vi "NotchFilterExample.vi"() -> ()   [LabVIEW 2011]
uses:
  <vilib>/addons/Digital Filter Design/_Objects.llb/DFD Filter Obj.ctl
  <vilib>/addons/Digital Filter Design/_Objects.llb/DFD Filter Coef.ctl
  <vilib>/addons/Digital Filter Design/_Objects.llb/DFD Filter Structure Type Selector.ctl
  <vilib>/addons/Digital Filter Design/_Objects.llb/dfd_Internal Quantization Settings.ctl
  <vilib>/addons/Digital Filter Design/_Objects.llb/dfd_Internal Quantization Srcs.ctl
  <vilib>/addons/Digital Filter Design/_Objects.llb/DFD Coef Norm Type.ctl
  <vilib>/Platform/TimedLoop/XDataNode/timing_clust.ctl
  <vilib>/Platform/TimedLoop/XDataNode/nitl_modes.ctl
  <vilib>/Platform/TimedLoop/XDataNode/wakeup.ctl
  <vilib>/addons/Digital Filter Design/Process.llb/DFD Filtering (PtByPt).vi
  <vilib>/addons/Digital Filter Design/Design.llb/DFD IIR Notch Peak Design by Q.vi
  <vilib>/measure/maspectr.llb/FFT Spectrum (Mag-Phase) for 1 Chan.vi
  <vilib>/Platform/TimedLoop/XDataNode/XDataNode.xnode
  <vilib>/addons/Digital Filter Design/NI_DigFilterLicensed.lvlib
  <vilib>/Platform/TimedLoop/XDataNode/XDNodeRunTimeDep.lvlib
  <vilib>/measure/NI_MAPro.lvlib
  <vilib>/Analysis/NI_AAL_SigProc.lvlib
panel:
  out "Waveform Graph":cluster{"f0":dbl, "df":dbl, "magnitude":dbl[]}(graph)
  out "Spectrum":T1(graph)={"magnitude"={"f0"=0.0, "df"=0.5, "magnitude"=array[500 elements]}, {"Locations"=[], "Amplitudes"=[]}}
  out "Peaks":cluster{"Locations":dbl[], "Amplitudes":dbl[]}
  out "FFTArray":dbl[](array[numeric])=[-5.97568735222049, -5.621732107397926, -5.038552645886518, -4.450468686097488, -4.0821691176339865, -4.0728882671460385, -4.423228798393417, -4.994943068826768, -5.563756411436293, -5.905055575012764, -5.8797121598680775, -5.4872592999993826, -4.866109771074623, -4.240732057590185, -3.8359611486272436, -3.791174228170831, -4.107113012463757, -4.6456645588715375, -5.182684017201283, -5.4936825586907805, -5.439650321745023, -5.020232627328567, -4.373947645235918, -3.7253620463457016, -3.2994014118795763, -3.2355255672229566, -3.53455059410871, -4.058429346991616, -4.583073945645599, -4.884043480291713, -4.822366769137059, -4.397718422044574, -3.7486363921120525, -3.0996975507319715, -2.67582805745418, -2.616478692364337, -2.9224469047901422, -3.455657403996944, -3.991984763648453, -4.3069412758428225, -4.2614998940832125, -3.855270518111671, -3.2267178015449245, -2.600337016849979, -2.2009647478759327, -2.167954576318933, -2.501999514596405, -3.0649130092321335, -3.632451984924015, -3.9800051633614593, -3.9684164942971876, -3.5971619499191885, -3.0045678614038747, -2.414987330139949, -2.053111481635458, -2.058145726336352, -2.430632777490008, -3.032234247915363, -3.63855429344588, -4.024828534809719, -4.051748093021613, -3.7186369869648788, -3.1636710696775863, -2.6110550334332903, -2.285334249334319, -2.3255716032657636, -2.732171076147873, -3.366659888069586, -4.004512671954646, -4.420840906380969, -4.476217440679121, -4.169854358986797, -3.639822357984511, -3.1102281666274734, -2.8055267719761563, -2.8646986114404758, -3.288073477970472, -3.93711295649828, -4.587234856114255, -5.013502866617332, -5.076451271616947, -4.775262964201894, -4.247988939226518, -3.7187257901481385, -3.411927974143003, -3.4665850057353715, -3.8830453254033332, -4.5227986616527796, -5.1613003513183635, -5.573660847179018, -5.6204702456554125, -5.30097608132646, -4.753302563210926, -4.2016277817257155, -3.8704956512435382, -3.898992749691152, -4.287571803114556, -4.897833635176491, -5.505351048003509, -5.8853578651631215, -5.8985729714374155, -5.544377597989529, -4.961034029931568, -4.372862267260028, -4.004551406249719, -3.9953359049822654, -4.3458184831566875, -4.917751478503985, -5.4868601285243965, -5.828531010742922, -5.8036354784589035, -5.411706343049822, -4.7911559821472816, -4.166452407081848, -3.7624300589685347, -3.7184654994695663, -4.035299748633417, -4.574819094338727, -5.112877844252291, -5.424986255538461, -5.372133481384279, -4.953963787254436, -4.308994218095225, -3.6617902515812126, -3.237276208462303, -3.1749105875042387, -3.475508078894869, -4.001020081877478, -4.527357198700525, -4.830076941127196, -4.770206489455651, -4.347418757702761, -3.700249946768749, -3.0532751211403877, -2.6314185804511787, -2.574129193616205, -2.8822024493396947, -3.4175610486766876, -3.9560775113904016, -4.273262031963773, -4.230085424554836, -3.8261554098870962, -3.1999344249714836, -2.575915490221136, -2.178932904134167, -2.1483379319809455, -2.4848212409065553, -3.050193905593625, -3.6202104546267977, -3.9702571916339395, -3.9611756287252606, -3.592439283228705, -3.0023720166497556, -2.4153244482992204, -2.0559852116514357, -2.0635572175870505, -2.438580674730889, -3.0427146886731977, -3.651560907900572, -4.040352448138856, -4.069777930226654, -3.739158880178784, -3.1866686679385774, -2.6365095149383793, -2.313224336133132, -2.355873578424281, -2.764858803333255, -3.401704833564521, -4.041883929062132, -4.460505222229892, -4.518139245370435, -4.213995797085913, -3.6861433223131272, -3.158686334338146, -2.856077642869327, -2.9172955484921985, -3.3426677500351385, -3.993653783142716, -4.645669454557922, -5.073776500704439, -5.138507302816345, -4.839042904548417, -4.3134325061869365, -3.785770963328159, -3.4805110538215676, -3.5366406731292472, -3.9545067046380984, -4.595597383365241, -5.235366617833823, -5.64892349920171, -5.696856830407549, -5.378412922075821, -4.831714830110095, -4.280939563913337, -3.9506300301078467, -3.979871873262168, -4.3691169614859104, -4.979965336896743, -5.5879890973503015, -5.9684214402525715, -5.98198070305598, -5.628047649102335, -5.044884175770395, -4.456809975924332, -4.08851391974228, -4.079230320581869, -4.429561835075211, -5.001260819724555, -5.570052612762078, -5.91132397441526, -5.885946522626465, -5.493453415206553, -4.872257457812066, -4.246827171079447, -3.8419975863494646, -3.7971459359695063, -4.11301399059333, -4.651488868014997, -5.188425784421577, -5.499335983347278, -5.445209681325951, -5.025692283231612, -4.379302048467413, -3.7306057431427964, -3.3045290492455734, -3.240531898371193, -3.539430483814445, -4.063177776836101, -4.587686019162704, -4.888514427985717, -4.826691953399974, -4.40189334194204, -3.752656688045358, -3.1035590089586815, -2.679526614489999, -2.620010439224742, -2.9258080910978457, -3.4588444419327233, -3.9949942317513787, -4.309769922651276, -4.264144641613878, -3.857728465171484, -3.2289862268718275, -2.602413382091327, -2.202846700372251, -2.169639951728965, -2.5034863393238003, -3.066199502682131, -3.6335365615561814, -3.980886434568021, -3.969093270084828, -3.5976332403932267, -3.00483287806273, -2.415045486969899, -2.0529623960081724, -2.057789219704304, -2.4300688758869358, -3.0314631822482, -3.637576499596384, -4.02364465351577, -4.050358969573484, -3.7170436706902104, -3.161874813225746, -2.60905729185776, -2.2831366789737193, -2.32317606042377, -2.7295796155764096, -3.363874761248236, -4.001536325176325, -4.417675978648588, -4.472866761392593, -4.166320945455444, -3.63610941273502, -3.106339074542322, -2.8014650972255586, -2.8604680942534175, -3.2836780312128524, -3.932556662080569, -4.582521961225087, -5.008637779789445, -5.071438558628105, -4.770107343809544, -4.242695278751824, -3.713299100894393, -3.4063734066835916, -3.460907845037558, -3.8772509858228417, -4.51689268178706, -5.155288388739395, -5.567548673021065, -5.614263739102609, -5.294681223971307, -4.746925433311064, -4.195174548350359, -3.8639725683239186, -3.8924061499761455, -4.280928092041427, -4.891139284660897, -5.498612590144155, -5.878581885895967, -5.891766104105767, -5.537546516874269, -4.9541854437162955, -4.366002912468052, -3.9976880406290696, -3.9884753008638563, -4.338967420792041, -4.9109167393786475, -5.4800484886628205, -5.821749234007299, -5.796890309851494, -5.405004502018551, -4.784504155913032, -4.159857243975239, -3.7558981618133718, -3.7120034189824933, -4.028913976874615, -4.568516058206815, -5.106663899035053, -5.418867678523341, -5.366116465536588, -4.948054434966055, -4.303198535018516, -3.656114140544593, -3.2317254634732495, -3.1694908878642893, -3.4702249834036305, -3.995879023159046, -4.522363477630227, -4.82523572140044, -4.765522792262976, -4.342897456551172, -3.6958957624356126, -3.049092616770561, -2.627412156802884, -2.5703030844570156, -2.87856071700568, -3.4141075797874505, -3.9528160127409544, -4.270196026570565, -4.2272182478951335, -3.823490206307066, -3.1974741442826664, -2.57366288447373, -2.1768905245989174, -2.1465081263058363, -2.483206150482008, -3.0487954631102827, -3.6190303818404144, -3.9692969973331236, -3.9604366069070593, -3.591922511482165, -3.002078354748901, -2.4152545370194805, -2.0561394717812216, -2.063935849176584, -2.439183656540288, -3.0435417778527367, -3.652611639873718, -4.041626136717718, -4.071273667942322, -3.740875538825938, -3.188604899345653, -2.6386637519522402, -2.3155947938232346, -2.358458255500911, -2.767655483787516, -3.4047110885148753, -4.0450971188268685, -4.463922498592392, -4.521757554071387, -4.217811880513517, -3.690153722402035, -3.162887395668834, -2.8604655159682792, -2.92186619332818, -3.34741693971202, -3.998577107777304, -4.650762325347665, -5.079034154185074, -5.143924805282298, -4.844615156665586, -4.319154247761323, -3.791636778258488, -3.486515375191596, -3.5427777884791163, -3.960770761371564, -4.601982394311398, -5.241866466948132, -5.655531947404552, -5.703567521554442, -5.385219389047899, -4.838610501030982, -4.287917768467314, -3.9576840059840306, -3.9869947726809474, -4.376301857830287, -4.987205231427335, -5.5952769260115325, -5.975750080536178, -5.989342980951666, -5.635436346098064, -5.052292035915185, -4.464229712933551, -4.095938224146738, -4.086651866909996, -4.436973289063696, -5.008654845550782, -5.577421880278855, -5.9186611664110185, -5.8932443420617195, -5.5007045924602895, -4.879454757897257, -4.253963400851944, -3.8490656016727236, -3.8041386488467386, -4.119924376259602, -4.658309971972454, -5.195150729418968, -5.505957976294024, -5.451722020134827, -5.032088363578573, -4.385575370471935, -3.7367499179437997, -3.310537805496792, -3.246399088612273, -3.545150090739972, -4.068743919441895, -4.593092958769223, -4.893756574130159, -4.831763869590888, -4.406789751268074, -3.757372478641705, -3.1080892393151047, -2.683866518592444, -2.6241554315480444, -2.929753771410782, -3.4625865999425915, -3.9985288515506543, -4.313093187001207, -4.267252936017326, -3.86061838176643, -3.2316545681211744, -2.6048571642713734, -2.2050631568561982, -2.171626536058367, -2.505240728073047, -3.067719598099761, -3.634820493999401, -3.981932564696965, -3.9699001908512184, -3.5981997787931608, -3.0051580966650997, -2.4151286852051976, -2.05280311124362, -2.057387228066914, -2.429424192864066, -3.0305760630449603, -3.636447439263071, -4.02227438683535, -4.048748470713145, -3.7151941526149286, -3.159787726873427, -2.6067343250881154, -2.2805797552619365, -2.3203873373422974, -2.7265614830242386, -3.360629839462558, -3.998067462499014, -4.4139862490763075, -4.468959461896693, -4.162199593072044, -3.6317777414407986, -3.1018010319062332, -2.7967248408464696, -2.855529987981699, -3.2785466411679898, -3.9272367524553355, -4.577018489899442, -5.002955893727491, -5.065583589099471, -4.764084801410969, -4.236510848247818, -3.7069586358754965, -3.399882924050603, -3.4542735193150205, -3.8704791433107615, -4.509989794548131, -5.148261068436077, -5.560403664611494, -5.607007914379096, -5.287321574979713, -4.7394690656276595, -4.187628674252066, -3.856344499821118, -3.884703291757965, -4.2731579343022466, -4.883309395838602, -5.4907306095679065, -5.870655516352556, -5.883803104333697, -5.5295546939854905, -4.94617264556551, -4.357977019957975, -3.98965695998956, -3.9804469558757862, -4.33094974499072, -4.902917668231767, -5.472075951743317, -5.813811147141563, -5.788994567287549, -5.397158968591169, -4.7767166592335935, -4.152135566639196, -3.7482500336439486, -3.7044365093125826, -4.021435886877789, -4.5611343132853746, -5.099385941260222, -5.411700859166119, -5.359068037653094, -4.941131546087548, -4.296408219919485, -3.6494633141250787, -3.22522091373631, -3.1631392690112645, -3.4640328090551007, -3.9898526596983963, -4.516509137684786, -4.819559457464254, -4.760030490468245, -4.337594830590808, -3.6907883476526084, -3.044185764403578, -2.6227110284212056, -2.565812646558062, -2.8742857358047464, -3.410052616195501, -3.9489854175373282, -4.266593935775643, -4.223848578348389, -3.8203566514517924, -3.194580170170159, -2.5710117259822614, -2.174485181869182, -2.1443513614181446, -2.481300484346546, -3.047143172605582, -3.6176334971707047, -3.96815729964722, -3.959555626137596, -3.5913015244452877, -3.0017183834839827, -2.4151563473790807, -2.0563035722724505, -2.064362490052009, -2.4398728291481406, -3.0444932142344032, -3.6538248126286494, -4.043100259105718, -4.0730076942598314, -3.742868165030517, -3.1908545639392134, -2.6411686371114507, -2.318352826802215, -2.361467110270621, -2.7709125829383634, -3.4082136054039247, -4.048841979980092, -4.467906386351882, -4.525976909488011, -4.222262906483061, -3.694832387037704, -3.1677894359227032, -2.865586441466155, -2.9272012904587474, -3.352961275923062, -4.004325536110784, -4.6567094891773175, -5.085174492182694, -5.150252556589672, -4.851124366266319, -4.325838772060686, -3.7984902908534193, -3.4935313728314927, -3.5499495972097552, -3.9680915428608214, -4.609445152340919, -5.249464054082875, -5.663257071803423, -5.7114127539526, -5.393177169875848, -4.8466731476768885, -4.296077482670671, -3.9659328813559305, -3.995324802342266, -4.384704942163973, -4.995673185928899, -5.603801489239893, -5.984322922157577, -5.997955709850103, -5.644080518574551, -5.060959163937324, -4.472911272459232, -4.104625663474488, -4.095336615091996, -4.445646764334581, -5.017308463788067, -5.586047063477411, -5.927249351164297, -5.901786988044713, -5.509193190897225, -4.8878808400194655, -4.262318546316348, -3.8573414469655356, -3.812326895626229, -4.128016799655316, -4.666298428822866, -5.203027166449752, -5.513714438202357, -5.459350657608405, -5.039581441210377, -4.392925274583408, -3.7439491642923217, -3.3175790468723445, -3.253275122308536, -3.551853865896033, -4.07526854424731, -4.599431707512776, -4.899902894114951, -4.8377113878678655, -4.412532281220043, -3.7629040263799887, -3.1134040099098668, -2.688958922104338, -2.6290200888701403, -2.9343855199168543, -3.4669804989229025, -4.002680187441947, -4.316997478398468, -4.270905938467135, -3.8640160923280105, -3.234793229704079, -2.607733269724446, -2.207673452834965, -2.1739680266301677, -2.507310678082698, -3.0695155362803326, -3.6363402158282607, -3.9831741349923915, -3.9708619461077195, -3.5988803292493037, -3.0055563281097992, -2.4152437605105157, -2.052634471621743, -2.05693459406838, -2.4286875650855086, -3.0295557225761476, -3.6351439478399756, -4.020688586738384, -4.046881484366051, -3.713047381922518, -3.1573628522749733, -2.6040333043349344, -2.277604821921041, -2.317140999021156, -2.7230465193284084, -3.356849299673936, -3.994024662996037, -4.409684770467747, -4.464403145907171, -4.157392539157608, -3.6267243031464567, -3.0965058129578074, -2.7911926910082596, -2.8497659986459287, -3.2725561407097237, -3.921025301338388, -4.570591875553075, -4.996320125185829, -5.05874489141586, -4.757049609847138, -4.229285802251864, -3.699550572844767, -3.3922988728836456, -3.446520693780551, -3.862564935205337, -4.50192176668307, -5.140046947428074, -5.552051333514287, -5.598525405144494, -5.278717060755513, -4.730750852909591, -4.178805194888971, -3.8474243028842556, -3.8756950352801813, -4.264070376900983, -4.874151388219596, -5.481511085936418, -5.8613834857098635, -5.874487641704263, -5.5202049315558455, -4.936797763754813, -4.348586238426562, -3.9802595285947824, -3.97105214558322, -4.321566838752948, -4.893555951835543, -5.462744704643959, -5.80451963329307, -5.779752025960149, -5.387974605214614, -4.767599636244794, -4.143094994375555, -3.739294961251586, -3.695575915723579, -4.012678671824875, -4.552489288389496, -5.090861821189817, -5.403306252876029, -5.350811439718738, -4.933021328131873, -4.288452622155449, -3.64167043700269, -3.2175987097330863, -3.155695534538873, -3.4567751765143084, -3.982788589682157, -4.509645911346777, -4.8129041690346686, -4.753590039961196, -4.331375916679908, -3.684797460742717, -3.0384291798894814, -2.6171948001528618, -2.560542600512994, -2.869267463977555, -3.4052914707033497, -3.944486504958051, -4.262362111724113, -4.219888442276495, -3.8166725417110077, -3.191176159309315, -2.5678916163153285, -2.171652501290262, -2.141809359484656, -2.47905212863597, -3.0451911453384284, -3.6159801921137626, -3.966804819295521, -3.9585057791819533, -3.590555823520937, -3.001278043215203, -2.4150222827031866, -2.056476397075878, -2.064842516083454, -2.4406600652373176, -3.0455873658074033, -3.6552252815218034, -4.044806143679235, -4.075017789811855, -3.7451809645083003, -3.1934682589557517, -2.644081119256466, -2.3215616892483006, -2.364969649689641, -2.7747058016973885, -3.4122942140715806, -4.053206400105752, -4.472550753557612, -4.530897076825501, -4.227454448091083, -3.7002906020735984, -3.1735093527719878, -2.8715628222288925, -2.933428635701005, -3.3594338297011093, -4.011037291249605, -4.663654192810659, -5.0923456515418986, -5.157643445038536, -4.858728029578418, -4.333648034930868, -3.806497763629879, -3.501729458488085, -3.55833049851534, -3.976647269769748, -4.618167529577204, -5.258344728926826, -5.672287522061034, -5.72058429610693, -5.402480967407508, -4.8561002195543015, -4.305618711992345, -3.975579024135332, -4.005066496447421, -4.394532716370502, -5.005577469109998, -5.613772619653975, -5.994351156853354, -6.008031234162517, -5.654193455702178, -5.071099584601804, -4.483069204628833, -4.114791102146382, -4.105499532119519, -4.455797118298613, -5.02743620988949, -5.596142163460768, -5.937301783231151, -5.911786756785091, -5.519130337201699, -4.897745450971697, -4.272100765056629, -3.8670314825139074, -3.821915032655541, -4.1374934082077734, -4.6756539739517695, -5.2122522177876665, -5.5227996794437555, -5.468286895882232, -5.048359616360676, -4.401536468318877, -3.752384609227775, -3.3258301354130193, -3.261333415413767, -3.559711101671834, -4.082916646386913, -4.606862793565731, -4.907109283575152, -4.844685610079926, -4.4192670830840335, -3.7693923798592297, -3.1196391193253943, -2.6949342312116835, -2.6347292877118065, -2.939822551440289, -3.4721395653593774, -4.007555756447308, -4.321584288924292, -4.275199006390161, -3.868010715804723, -3.238484994261437, -2.611118053069307, -2.210747429385189, -2.1767276717592328, -2.509752772075492, -3.0716371679895413, -3.6381387860353214, -3.9846473594706087, -3.972007858364352, -3.59969728297488, -3.0060429993000004, -2.4153991492892866, -2.052457903732966, -2.056425722052905, -2.4278463691412373, -3.0283825110907063, -3.6336393576025925, -4.018853582826432, -4.044717359710772, -3.710555756543763, -3.154545672199507, -2.6008928401790263, -2.2741436671689947, -2.3133620679642286, -2.718953044691952, -3.352444829926184, -3.9893130593393855, -4.404670203516313, -4.459090092055842, -4.151785776638609, -3.6208289077881464, -3.0903271536385093, -2.7847364248089512, -2.8430380657250605, -3.2655627588731146, -3.9137729603433873, -4.563087331115283, -4.988570392737175, -5.050757239572912, -4.74883155363896, -4.220845096076847, -3.690895203197259, -3.383437050825514, -3.4374608471836794, -3.8533157007721766, -4.492491981741846, -5.130445641521714, -5.542287719783991, -5.588608871518526, -5.268657160952961, -4.720557297266353, -4.168487841006326, -3.836993146135313, -3.865160199146582, -4.253442103179915, -4.863440027090745, -5.470727085912743, -5.850537383471874, -5.863590051832546, -5.5092665361680115, -4.925829302064603, -4.337598496226178, -3.969263327670066, -3.960058333090827, -4.310586276539543, -4.882599505740745, -5.451823233765801, -5.793643979257983, -5.768933002188373, -5.377222986193022, -4.7569261468257755, -4.132510299106359, -3.728809653747007, -3.6852005080893075, -4.002423584150208, -4.542364838307881, -5.080878213534376, -5.3934735694132305, -5.341139629004578, -4.923520195475749, -4.279131819709457, -3.632539453988619, -3.208666862813941, -3.1469719583453366, -3.4482688143389457, -3.974508184342159, -4.501599996237134, -4.805101059369049, -4.746037824217132, -4.324082448255902, -3.6777703498249843, -3.0316757855645227, -2.6107222227324143, -2.5543576741248213, -2.8633767493898525, -3.399701248422441, -3.9392027685767923, -4.257390561555547, -4.2152344792644305, -3.812341261621601, -3.1871723472206854, -2.564219741402525, -2.16831671191447, -2.138813478592101, -2.4763996494699243, -3.042885227469357, -3.614023657801723, -3.9652001501612086, -3.9572551132284013, -3.589660952477597, -3.0007404102273916, -2.4148429803563762, -2.0566561657660607, -2.0653817427316, -2.441558782353785, -3.046845250899329, -3.656841656854458, -4.046779976392003, -4.077347692371797, -3.7478651955301725, -3.196504724357843, -2.6474673737838823, -2.3252949383300954, -2.3690467516490394, -2.7791232703123723, -3.417048221474208, -4.0582927800265045, -4.47796500490699, -4.536634367616659, -4.233509619687866, -3.706658173776228, -3.180183526715912, -2.8785374886233335, -2.9406973783658517, -3.366989931923136, -4.018873741943371, -4.671763692986944, -5.100720621052456, -5.1662760296299375, -4.867610108213487, -4.342771227393865, -3.815853438392654, -3.5113087408417716, -3.5681242789522942, -3.9866462126102125, -4.6283620818400975, -5.268725129412937, -5.6828438106784125, -5.731306323384437, -5.413358404229662, -4.867122567072562, -4.316775311735933, -3.9868590682825973, -4.016459038264088, -4.406026680806378, -5.017161663533356, -5.625435744721792, -6.006081817503519]
  in  "ChartLength":dbl=2000.0
  out "Notch":T2={"mSRate_Fs"=1000.0, "mSRate_Version"="2.0", "mSRate_Comments"="", "mSRate_OrgCoef"={"type"=enum."IIR Direct Form II", "gain"=1.0, "coef a (k)"=[1.0, -1.9974443312996026, 0.9984304360830942], "coef b (v)"=[0.9992152180415471, -1.9974443312996026, 0.9992152180415471]}, "mSRate_CurCoef"={"type"=enum."IIR Direct Form II", "gain"=1.0, "coef a (k)"=[1.0, -1.9974443312996026, 0.9984304360830942], "coef b (v)"=[0.9992152180415471, -1.9974443312996026, 0.9992152180415471]}, "mSRate_Quantized?"=FALSE, "mSRate_QCoef"={"type"=enum."Undefined", "gain"=1.0, "coef a (k)"=[], "coef b (v)"=[]}, "mSRate_QSettings"=[], "mSRate_Order"=2, "mSRate_Scaling"={"mSRate_ScaleByPowerOf2?"=FALSE, "mSRate_ScaleType"=enum."No Norm"}} {"mSRate_QSettings"."source" items=["Coef a/k"=0, "Coef b/v"=7, "Input"=1, "Output"=2, "Multiplicand"=3, "Product"=4, "Sum"=5, "Delay"=6, "Gain"=8]}
  in  "Q":dbl=20.0 format="%.2f"
  in  "SigFreq(Hz)":dbl=10.0
  out "Finished Late? [i-1]":bool
  out "Waveform Chart":cluster{dbl, "signal out":dbl}(graph)={-1.943171217609549, "signal out"=-5.97568735222049}
  in  "stop":bool
  in  "NotchFreq(Hz)":dbl=5.0 format="%.2f"
  in  "LoopFreq(Hz)":dbl=1000.0 caption="Set Loop Period (us)"
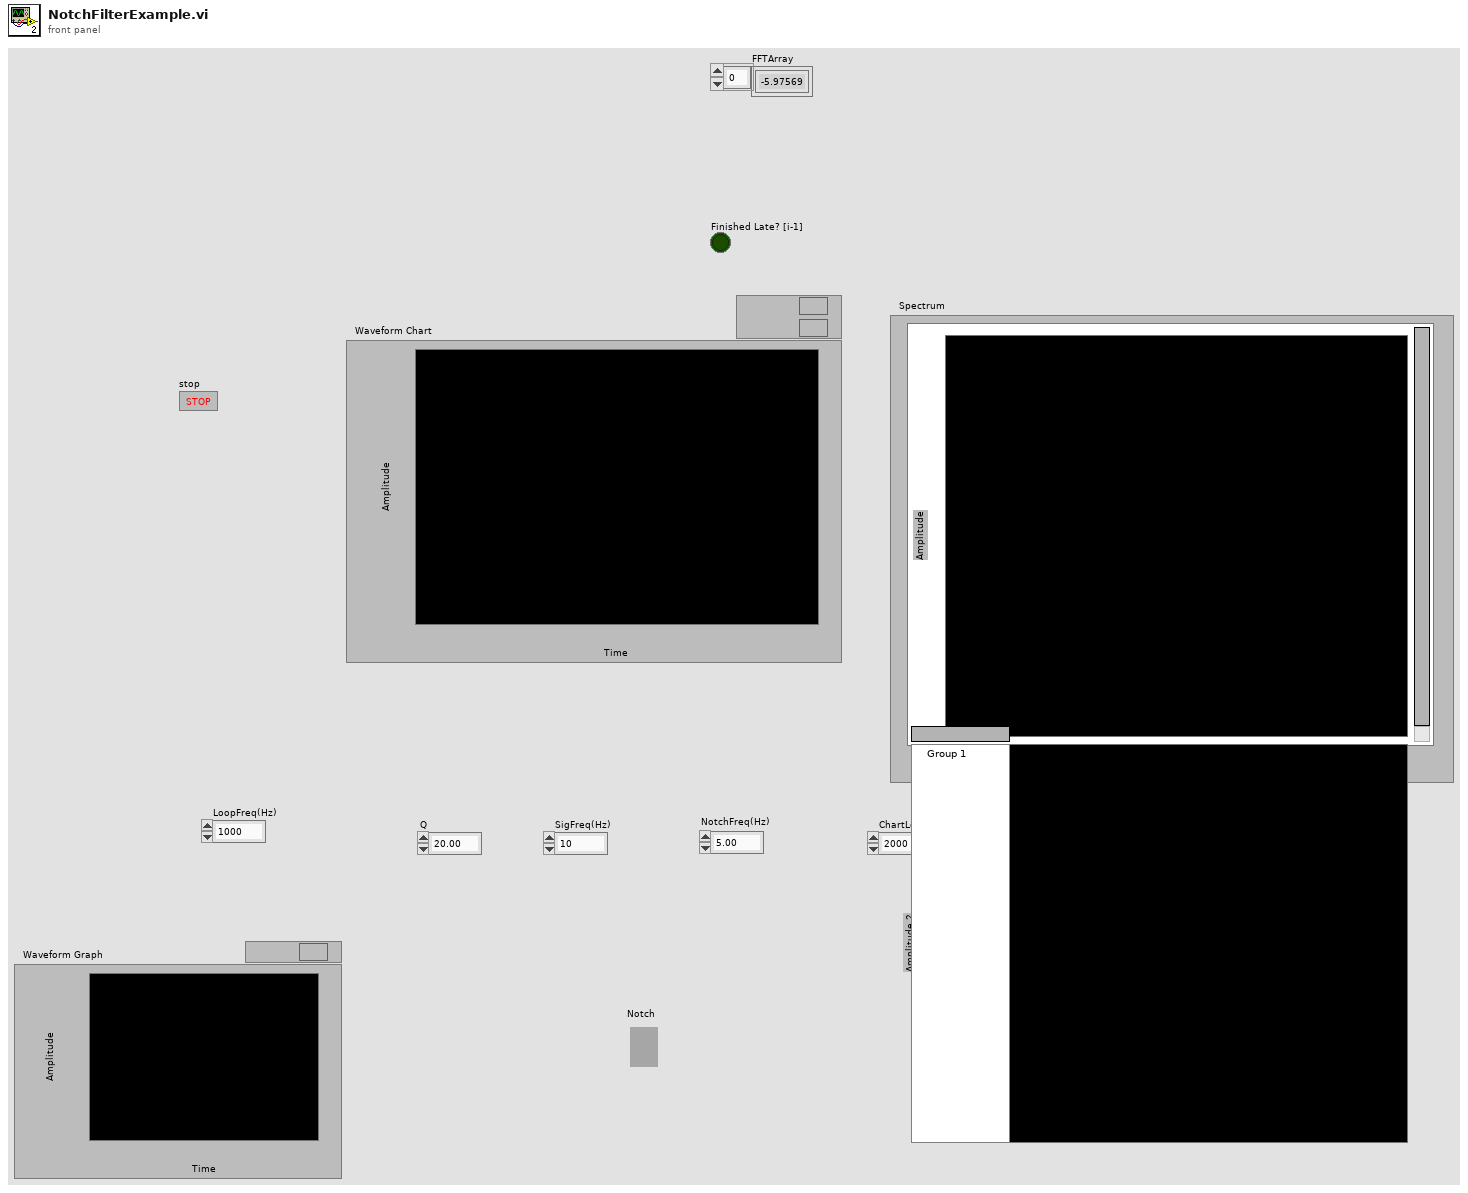
[diagram p1: front panel]
types:
  T1 = cluster{"magnitude":cluster{"f0":dbl, "df":dbl, "magnitude":dbl[]}, cluster{"Locations":dbl[], "Amplitudes":dbl[]}}
  T2 = typedef "NI_DigFilterLicensed.lvlib/DFD Filter Obj.ctl" = cluster{"mSRate_Fs":dbl, "mSRate_Version":string, "mSRate_Comments":string, "mSRate_OrgCoef":T3, "mSRate_CurCoef":T3, "mSRate_Quantized?":bool, "mSRate_QCoef":T3, "mSRate_QSettings":T5[], "mSRate_Order":i32, "mSRate_Scaling":cluster{"mSRate_ScaleByPowerOf2?":bool, "mSRate_ScaleType":T7}}
  T3 = typedef "NI_DigFilterLicensed.lvlib/DFD Filter Coef.ctl" = cluster{"type":T4, "gain":dbl, "coef a (k)":dbl[], "coef b (v)":dbl[]}
  T4 = typedef "NI_DigFilterLicensed.lvlib/DFD Filter Structure Type Selector.ctl" = enum16{"Undefined", "FIR Direct Form", "FIR Direct Form Transposed", "FIR Symmetric", "FIR Antisymmetric", "IIR Direct Form I", "IIR Direct Form I Transposed", "IIR Direct Form II", "IIR Direct Form II Transposed", "IIR Cascaded Second Order Sections Form I", "IIR Cascaded Second Order Sections Form I Transposed", "IIR Cascaded Second Order Sections Form II", "IIR Cascaded Second Order Sections Form II Transposed", "Lattice Allpass (basic sections)", "Lattice Allpass (one multiplier sections)", "Lattice Allpass (normalized sections)", "Lattice AR (basic sections)", "Lattice AR (one multiplier sections)", "Lattice AR (normalized sections)", "Lattice MA (minimum phase)", "Lattice MA (maximum phase)", "Lattice ARMA (basic sections)", "Lattice ARMA (one multiplier sections)", "Lattice ARMA (normalized sections)"}
  T5 = typedef "NI_DigFilterLicensed.lvlib/dfd_Internal Quantization Settings.ctl" = cluster{"source":T6, "wl":i16, "iwl":i16, "overflow mode":enum16{"Saturation", "Wrap"}, "rounding mode":enum16{"Nearest", "Truncation"}, "signed?":bool}
  T6 = typedef "NI_DigFilterLicensed.lvlib/dfd_Internal Quantization Srcs.ctl" = u16
  T7 = typedef "NI_DigFilterLicensed.lvlib/DFD Coef Norm Type.ctl" = enum16{"No Norm", "Time Domain 1-Norm", "Time Domain 2-Norm", "Time Domain Inf-Norm"}
  T8 = typedef "XDNodeRunTimeDep.lvlib/timing_clust.ctl" = cluster{"Expected End [f-1]":u64, "Actual End [f-1]":u64, "Finished Late? [f-1]":bool, "Expected End [i-1]":u64, "Actual End [i-1]":u64, "Finished Late? [i-1]":bool, "Expected Start [i]":u64, "Actual Start [i]":u64, "Expected Start [f]":u64, "Actual Start [f]":u64, "Source Name":string, "Structure Name":string, "Period":i64, "Deadline":i64, "Offset":i64, "Start":i64, "Priority":i32, "Timeout":i32, "Mode":T9, "Wakeup Reason":T10, "Error":errorcluster, "Source Type":string, "Secondary Source Type":string, "Global End Time":u64, "Global Start Time":u64, "Frame Duration":u64, "Iteration Duration":u64, "Assigned CPU":i32, "I/O Scan Engine Mode":u32}
  T9 = typedef "XDNodeRunTimeDep.lvlib/nitl_modes.ctl" = enum32{"No Change", "Process missed periods, maintain original phase", "Discard missed periods, maintain original phase", "Process missed periods, ignore original phase", "Discard missed periods, ignore original phase"}
  T10 = typedef "XDNodeRunTimeDep.lvlib/wakeup.ctl" = enum32{"Normal", "Aborted", "Asynchronous wakeup", "Timing source error", "Timed loop error", "Timeout"}
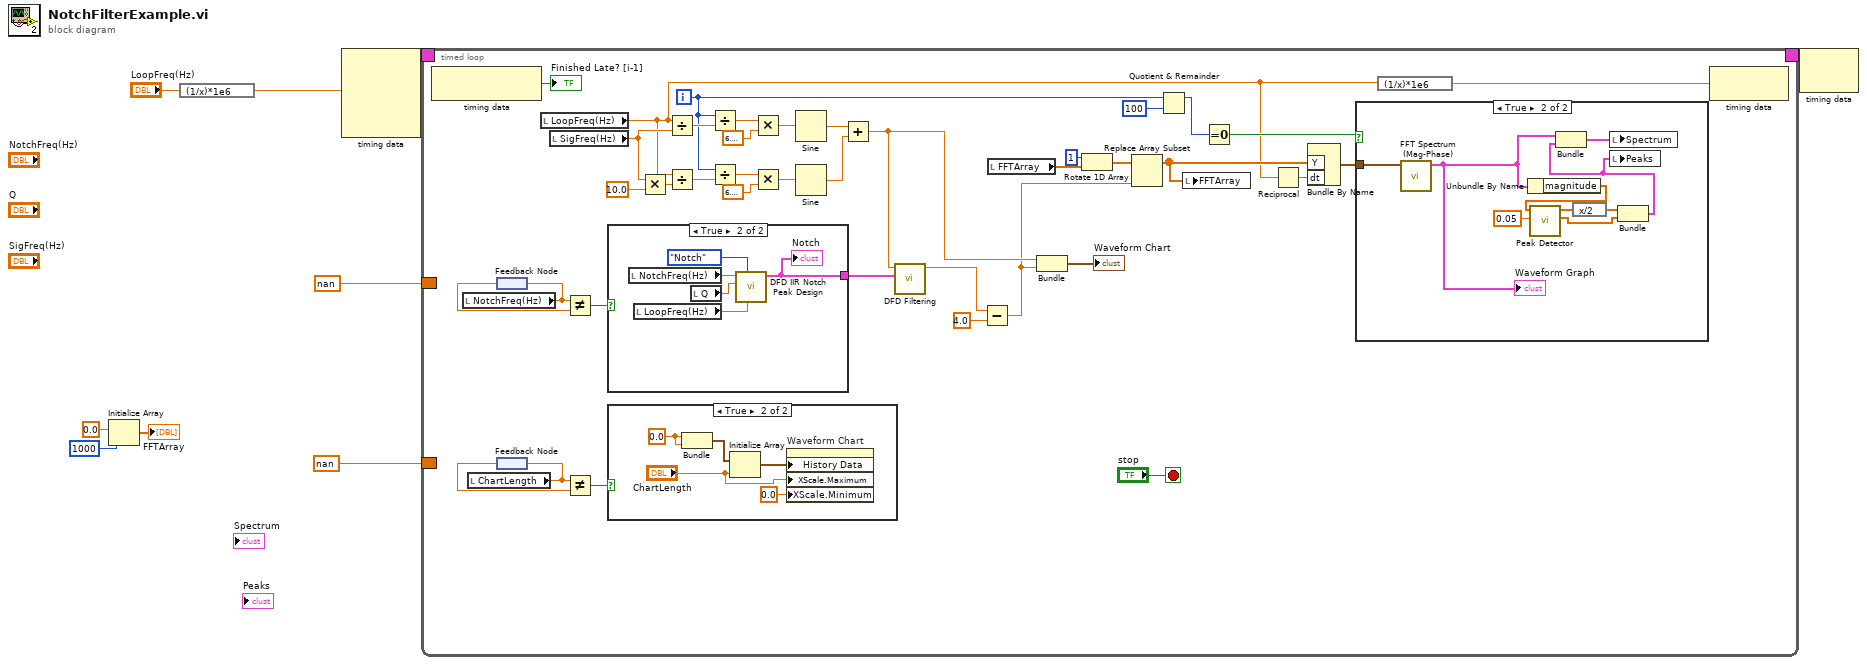
[diagram p0: block diagram]
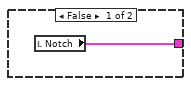
[diagram p4: hidden frame]
diagram:
  n1 = Initialize Array(0.0, 1000 ("dimension size")) -> (→"FFTArray":dbl[])
  n2 = expression code="(1/x)*1e6"("LoopFreq(Hz)") -> (w6:dbl)
  n3 = node-c288(w6) -> (w9:T8)  [unwired: 3 in]
  n4 = timed-loop {
    timing: w9 -> [_]
    timing-out: [_] -> w8
    border: nan ("NotchFreq(Hz)") -> [_]
    border: nan ("LoopFreq(Hz)") -> [_]
    i -> [w19]
    stop <- "stop" stop-if-true
    n5 = node-c288() -> (→"Finished Late? [i-1]":bool)  [unwired: 1 in]
    n6 = local read "NotchFreq(Hz)"() -> (w41:dbl)
    n7 = local read "ChartLength"() -> (w25:dbl)
    n8 = feedback-in #1(w41) -> ()
    n9 = feedback #1() -> (w40:dbl)
    n10 = feedback #2() -> (w26:dbl)
    n11 = feedback-in #2(w25) -> ()
    n12 = local read "LoopFreq(Hz)"() -> (w10:dbl)
    n13 = local read "SigFreq(Hz)"() -> (w33:dbl)
    n14 = Not Equal?(x=w41, y=w40) -> (x != y?=w42:bool)
    n15 = Not Equal?(x=w25, y=w26) -> (x != y?=w24:bool)
    n16 = case shown="True" w42 {
      tunnel: [w63 w64] -> w39
      frame False {
        n17 = local read "Notch"() -> (w63:T2)
      }
      frame True {
        n18 = local read "NotchFreq(Hz)"() -> (w67:dbl)
        n19 = local read "LoopFreq(Hz)"() -> (w66:dbl)
        n20 = local read "Q"() -> (w65:dbl)
        n21 = call-poly <vilib>:"DFD IIR Notch Peak Design.vi"("fs [Hz]"=w66, "filter type"=enum16{"Notch", "Peak"}."Notch", "Q factor"=w65, "f0 [Hz]"=w67) -> ("filter out"=w64:T2)  [unwired: 1 in, 6 out]
        "Notch" <- w64
      }
    }
    n22 = case shown="True" w24 {
      frame False {
      }
      frame True {
        w60 = 0.0 ("element")
        n23 = Bundle("element"=w60, "element"=w60) -> (w61:cluster{"element":dbl, "element":dbl})  [unwired: 1 in]
        n24 = Initialize Array(w61, "ChartLength") -> (w62:cluster{"element":dbl, "element":dbl}[])
        n25 = property on="Waveform Chart" class="WFChart (strict)"("History Data"=w62, "XScale.Maximum"="ChartLength", "XScale.Minimum"=0.0 ("X Scale.Range:Minimum")) -> ()  [unwired: 2 in, 2 out]
      }
    }
    n26 = Multiply(x=w33, y=10.0) -> (x*y=w34:dbl)
    n27 = Divide(x=w10, y=w33) -> (x/y=w43:dbl)
    n28 = Divide(x=w10, y=w34) -> (x/y=w38:dbl)
    n29 = Divide(x=w19, y=w43) -> (x/y=w48:dbl)
    n30 = Divide(x=w19, y=w38) -> (x/y=w35:dbl)
    n31 = Multiply(x=w48, y=6.283185307179586) -> (x*y=w45:dbl)
    n32 = Multiply(x=w35, y=6.283185307179586) -> (x*y=w37:dbl)
    n33 = Sine(x=w45) -> (sin(x)=w31:dbl)
    n34 = Sine(x=w37) -> (sin(x)=w30:dbl)
    n35 = Add(x=w31, y=w30) -> (x+y=w21:dbl)
    n36 = call-poly <vilib>:"DFD Filtering.vi"("filter"=w39, "signal in"=w21) -> ("signal out"=w29:dbl)  [unwired: 2 in, 7 out]
    n37 = Subtract(x=w29, y=4.0) -> (x-y=w15:dbl)
    n38 = local read "FFTArray"() -> (w23:dbl[])
    n39 = Bundle(w21, w15) -> (→"Waveform Chart":cluster{dbl, dbl})  [unwired: 1 in]
    n40 = Rotate 1D Array(1:w23, 2:1 ("n")) -> (0:w20:dbl[])
    n41 = Replace Array Subset(array=w20, new element=w15) -> (w14:dbl[])  [unwired: 1 in]
    n42 = Quotient & Remainder(x=w19, y=100) -> (x-y*floor(x/y)=w17:i32)  [unwired: 1 out]
    n43 = local write "FFTArray"(w14) -> ()
    n44 = Equal To 0?(x=w17) -> (x = 0?=w16:bool)
    n45 = Reciprocal(x=w10) -> (1/x=w11:dbl)
    n46 = Bundle By Name("Y"=w14, "dt"=w11) -> (w12:waveform(dbl))  [unwired: 1 in]
    n47 = case shown="True" w16 {
      tunnel: w12 -> [_ w50]
      frame False {
      }
      frame True {
        n48 = call-poly <vilib>:"FFT Spectrum (Mag-Phase).vi"("time signal"=w50) -> ("magnitude"=w49:cluster{"f0":dbl, "df":dbl, "magnitude":dbl[]})  [unwired: 6 in, 4 out]
        "Waveform Graph" <- w49
        n49 = Unbundle By Name(w49) -> ("magnitude"=w51:dbl[])
        n50 = call <vilib>:"Peak Detector.vi"("threshold"=0.05, "X"=w51) -> ("Amplitudes"=w53:dbl[], "Locations"=w54:dbl[])  [unwired: 5 in, 3 out]
        n51 = expression code="x/2"(w54) -> (w55:dbl[])
        n52 = Bundle("Locations"=w55, "Amplitudes"=w53) -> (w56:cluster{"Locations":dbl[], "Amplitudes":dbl[]})  [unwired: 1 in]
        n53 = Bundle("magnitude"=w49, w56) -> (w57:T1)  [unwired: 1 in]
        n54 = local write "Spectrum"(w57) -> ()
        n55 = local write "Peaks"(w56) -> ()
      }
    }
    n56 = expression code="(1/x)*1e6"(w10) -> (w13:dbl)
    n57 = node-c288(w13) -> ()  [unwired: 1 out]
  }
  n58 = node-c288(w8) -> ()  [unwired: 1 out]
